vi "test.vi"() -> ()   [LabVIEW 2014]
uses:
  <vilib>/measure/maresamp.llb/Align two Waveforms (continuous).vi
  <vilib>/express/express analysis/Spectral/Block/exnSpectralBlock spectral measurements peak poly.vi
  <vilib>/express/express analysis/Spectral/Block/exnSpectralBlock spectral measurements peak DDT.vi
  <vilib>/express/express analysis/Spectral/XNode/ExpressSpectralMeasurementsBlockNode.xnode
  <vilib>/measure/NI_MAPro.lvlib
panel:
  out "Phase Difference":dbl=-4.668681158228912
  in  "Upper Cut-Off 2":dbl=12500.0 caption="Upper Cut-Off"
  in  "Upper Cut-Off":dbl=15000.0
  in  "Lower Cut-Off 2":dbl=4000.0 caption="Lower Cut-Off"
  in  "Lower Cut-Off":dbl=4000.0
  out "Demodulated R(t) Signal":dynamicdata(graph)=[{"t0"=timestamp(0 s since 1904-01-01), "dt"=2.2727272727272728e-06, "Y"=array[43991 elements], "attributes"=variant("NI_ChannelName"=variant(string "Filtered (Filtered)"), "NI_OriginalChannelName"=variant(string "Filtered"))}] caption="Filtered Signal"
  out "Demodulated I(t) Signal":dynamicdata(graph)=[{"t0"=timestamp(0 s since 1904-01-01), "dt"=2.2727272727272728e-06, "Y"=array[43991 elements], "attributes"=variant("NI_ChannelName"=variant(string "Filtered (Filtered)"), "NI_OriginalChannelName"=variant(string "Filtered"))}] caption="Filtered Signal"
  out "FFT of R(t)":dynamicdata(graph)=[{"t0"=timestamp(0 s since 1904-01-01), "dt"=10.002045873019481, "Y"=array[21996 elements], "attributes"=variant("NI_ChannelName"=variant(string "Filtered (FFT - (Peak))"), "NI_OriginalChannelName"=variant(string "Filtered"))}]
  out "FFT of I(t)":dynamicdata(graph)=[{"t0"=timestamp(0 s since 1904-01-01), "dt"=10.002045873019481, "Y"=array[21996 elements], "attributes"=variant("NI_ChannelName"=variant(string "Filtered (FFT - (Peak))"), "NI_OriginalChannelName"=variant(string "Filtered"))}]
  out "Transmitted Composit Signal":waveform(dbl)(graph)={"t0"=timestamp(3 s since 1904-01-01), "dt"=2.2727272727272728e-06, "Y"=array[44000 elements], "attributes"=variant("NI_ChannelName"=variant(string "Sine"), "NI_ExpIsRelativeTime"=variant(bool TRUE), "NI_ExpStartTimeStamp"=variant(timestamp timestamp(3501202748.2762866 s since 1904-01-01)), "NI_ExpTimeStamp"=variant(timestamp timestamp(3501202751.2762866 s since 1904-01-01)), "NI_ExpXDimension"=variant(string "t"))}
  in  "I(t) Frequency":dbl=7000.0 caption="Frequency"
  in  "I(t) Amplitude":dbl=1.0 caption="Amplitude"
  in  "R(t) Frequency":dbl=5000.0 caption="Frequency"
  in  "R(t) Amplitude":dbl=1.0 caption="Amplitude"
  out "Modulated signals":waveform(dbl)[](graph)=[{"t0"=timestamp(3 s since 1904-01-01), "dt"=2.2727272727272728e-06, "Y"=array[44000 elements], "attributes"=variant("NI_ChannelName"=variant(string "Sine"), "NI_ExpIsRelativeTime"=variant(bool TRUE), "NI_ExpStartTimeStamp"=variant(timestamp timestamp(3501202748.2762866 s since 1904-01-01)), "NI_ExpTimeStamp"=variant(timestamp timestamp(3501202751.2762866 s since 1904-01-01)), "NI_ExpXDimension"=variant(string "t"))}, {"t0"=timestamp(3 s since 1904-01-01), "dt"=2.2727272727272728e-06, "Y"=array[44000 elements], "attributes"=variant("NI_ChannelName"=variant(string "Sine"), "NI_ExpIsRelativeTime"=variant(bool TRUE), "NI_ExpStartTimeStamp"=variant(timestamp timestamp(3501202748.2762866 s since 1904-01-01)), "NI_ExpTimeStamp"=variant(timestamp timestamp(3501202751.2762866 s since 1904-01-01)), "NI_ExpXDimension"=variant(string "t"))}]
  out "Carrier":waveform(dbl)[](graph)=[{"t0"=timestamp(3 s since 1904-01-01), "dt"=2.2727272727272728e-06, "Y"=array[44000 elements], "attributes"=variant("NI_ChannelName"=variant(string "Sine"), "NI_ExpIsRelativeTime"=variant(bool TRUE), "NI_ExpStartTimeStamp"=variant(timestamp timestamp(3501202748.2762866 s since 1904-01-01)), "NI_ExpTimeStamp"=variant(timestamp timestamp(3501202751.2762866 s since 1904-01-01)), "NI_ExpXDimension"=variant(string "t"))}, {"t0"=timestamp(3 s since 1904-01-01), "dt"=2.2727272727272728e-06, "Y"=array[44000 elements]}]
  in  "Carrier Amplitude":dbl=1.0 caption="Amplitude"
  in  "Carrier Frequency":dbl=10000.0 caption="Frequency"
  in  "Carrier Amplitude 2":dbl=1.0 caption="Amplitude"
  in  "Carrier Frequency 2":dbl=10000.0 caption="Frequency"
  in  "stop 2":bool
  out "data":dynamicdata(graph)=[{"t0"=timestamp(3501202754.2033076 s since 1904-01-01), "dt"=1.1109999999999994e-05, "Y"=array[9000 elements], "attributes"=variant("NI_ChannelName"=variant(string "Voltage"), "NI_UnitDescription"=variant(string "Volts"))}] caption="Received Signal"
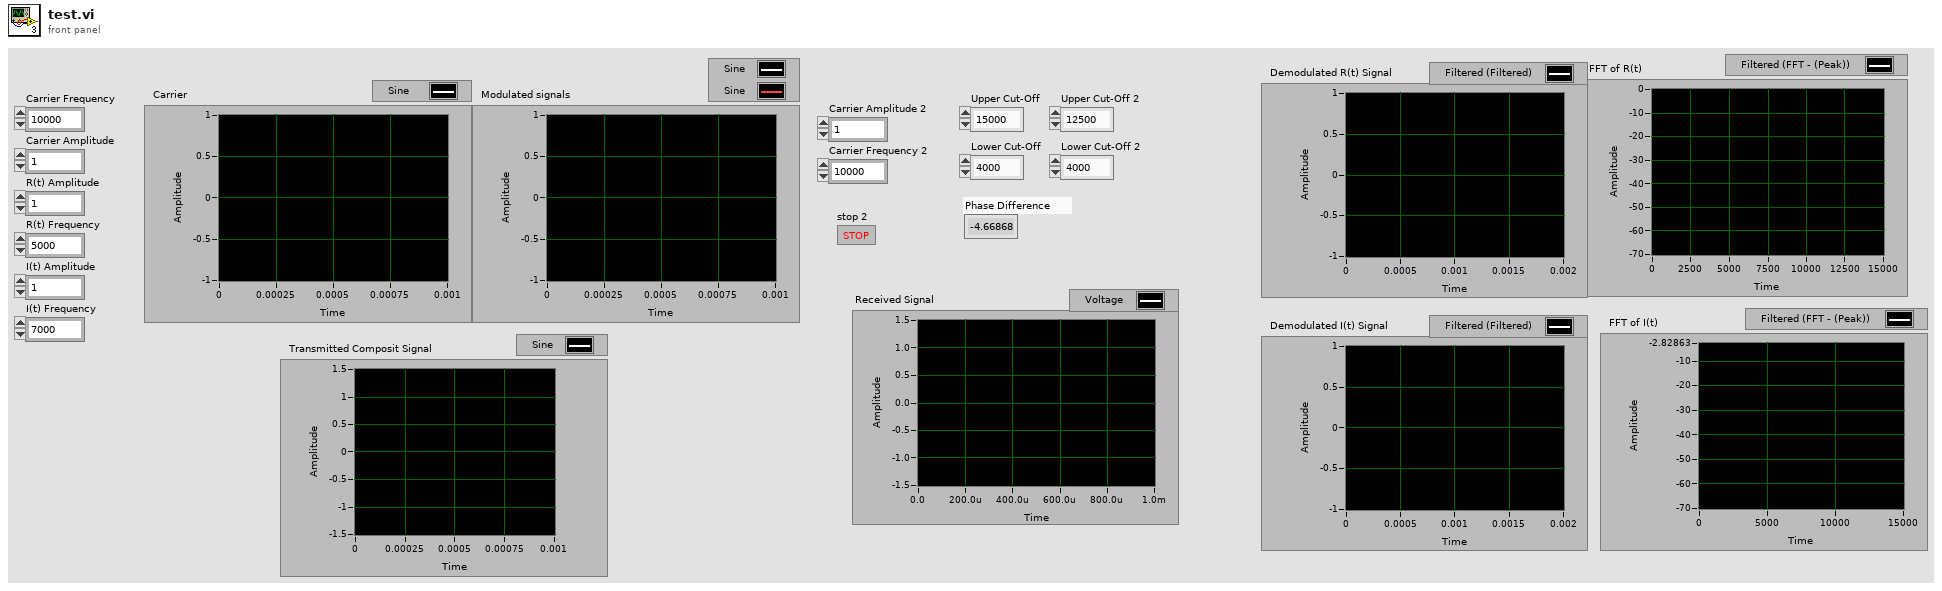
[diagram p1: front panel]
types:
  T1 = cluster{"averaging mode":u16, "weighting mode":u16, "number of averages":u32}
  T2 = cluster{"dB On (F)":bool, "unwrap phase (F)":bool, "convert to degree (F)":bool}
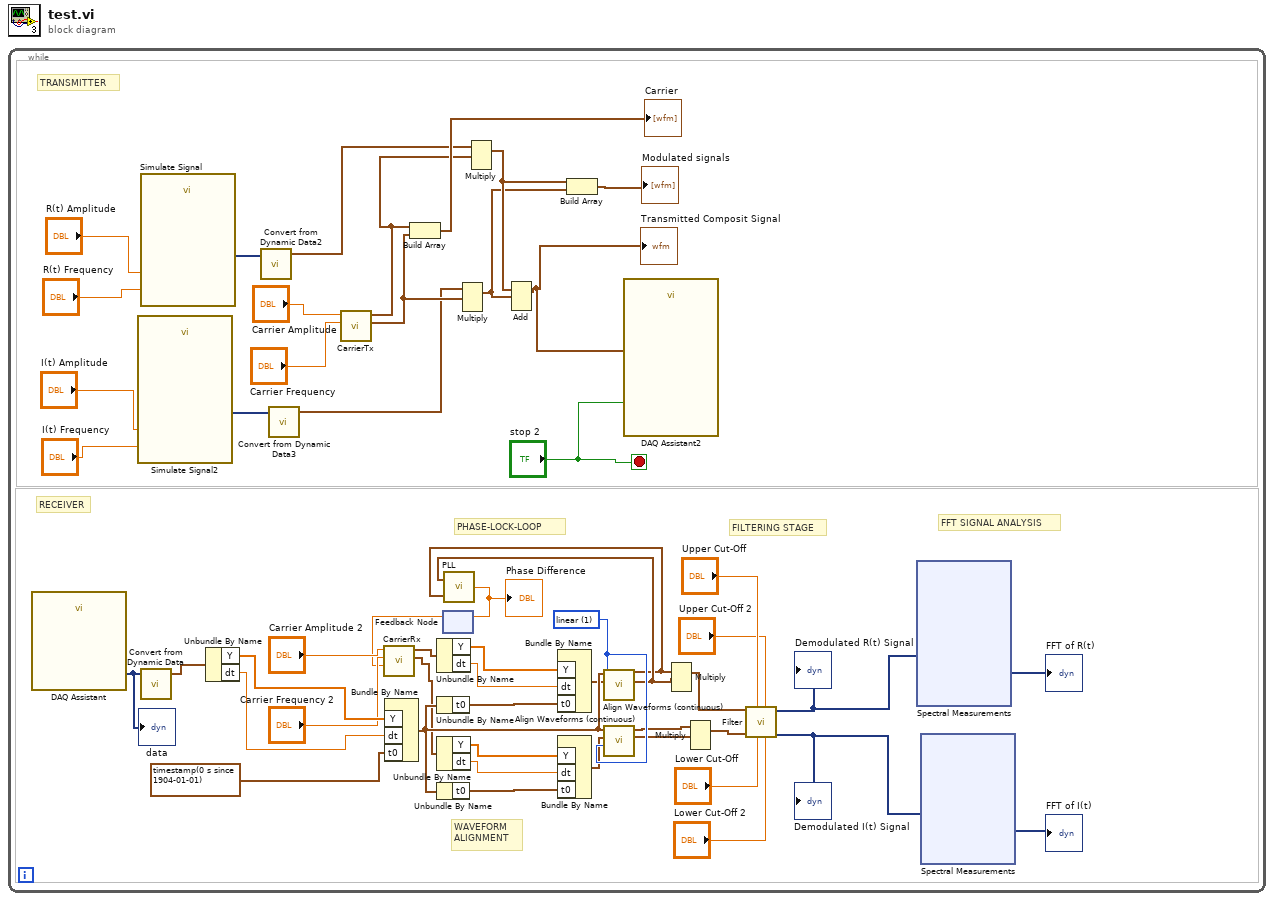
[diagram p0: block diagram]
diagram:
  n1 = while {
    stop <- "stop 2" stop-if-true
    w43 = u16 1 items=["coerce", "linear", "spline", "FIR filter"] ("interpolation mode")
    # "FFT SIGNAL ANALYSIS"
    # "FILTERING STAGE"
    # "PHASE-LOCK-LOOP"
    # "WAVEFORM\nALIGNMENT"
    # "RECEIVER"
    # "TRANSMITTER"
    n2 = call "DAQ Assistant"() -> ("data"=w53:dynamicdata)  [unwired: 17 in, 2 out]
    "data" <- w53
    n3 = call "Simulate Signal2"("Frequency"="I(t) Frequency", "Amplitude"="I(t) Amplitude") -> ("Sine"=w34:dynamicdata)  [unwired: 12 in, 1 out]
    n4 = call "Simulate Signal"("Frequency"="R(t) Frequency", "Amplitude"="R(t) Amplitude") -> ("Sine"=w39:dynamicdata)  [unwired: 12 in, 1 out]
    n5 = call "Convert from Dynamic Data"("Dynamic Data Type"=w53) -> ("Waveform"=w8:waveform(dbl))  [unwired: 3 in]
    n6 = Unbundle By Name(w8) -> ("Y"=w51:dbl[], "dt"=w50:dbl)
    n7 = call "Convert from Dynamic Data2"("Dynamic Data Type"=w39) -> ("Waveform"=w38:waveform(dbl))  [unwired: 3 in]
    n8 = call "Convert from Dynamic Data3"("Dynamic Data Type"=w34) -> ("Waveform"=w31:waveform(dbl))  [unwired: 3 in]
    n9 = call "CarrierTx.vi"("Carrier Frequency"="Carrier Frequency", "Carrier Amplitude"="Carrier Amplitude") -> ("I(t) Carrier"=w32:waveform(dbl), "R(t) Carrier"=w37:waveform(dbl))  [unwired: 8 in]
    n10 = Bundle By Name("Y"=w51, "dt"=w50, "t0"=timestamp(0 s since 1904-01-01)) -> (w44:waveform(dbl))  [unwired: 1 in]
    n11 = Build Array(w37, w32) -> (→"Carrier":waveform(dbl)[])
    n12 = Unbundle By Name(w44) -> ("t0"=w47:timestamp)
    n13 = Unbundle By Name(w44) -> ("t0"=w45:timestamp)
    n14 = feedback #1() -> (w18:dbl)  [unwired: 1 in]
    n15 = call "CarrierRx.vi"("Phase"=w18, "Carrier Frequency"="Carrier Frequency 2", "Carrier Amplitude"="Carrier Amplitude 2") -> ("I(t) Carrier"=w20:waveform(dbl), "R(t) Carrier"=w7:waveform(dbl))  [unwired: 7 in]
    n16 = Unbundle By Name(w7) -> ("Y"=w49:dbl[], "dt"=w48:dbl)
    n17 = Unbundle By Name(w20) -> ("Y"=w29:dbl[], "dt"=w46:dbl)
    n18 = Multiply(1:w32, 2:w31) -> (0:w24:waveform(dbl))  [unwired: 1 in, 1 out]
    n19 = Multiply(1:w37, 2:w38) -> (0:w25:waveform(dbl))  [unwired: 1 in, 1 out]
    n20 = Add(1:w24, 2:w25) -> (0:w26:waveform(dbl))  [unwired: 1 in, 1 out]
    "Transmitted Composit Signal" <- w26
    n21 = Bundle By Name("Y"=w49, "dt"=w48, "t0"=w47) -> (w27:waveform(dbl))  [unwired: 1 in]
    n22 = Bundle By Name("Y"=w29, "dt"=w46, "t0"=w45) -> (w28:waveform(dbl))  [unwired: 1 in]
    n23 = Build Array(w25, w24) -> (→"Modulated signals":waveform(dbl)[])
    n24 = call-poly <vilib>:"Align Waveforms (continuous).vi"("interpolation mode"=w43, "waveform B in"=w27, "waveform A in"=w44) -> ("waveform B out"=w6:waveform(dbl), "waveform A out"=w3:waveform(dbl))  [unwired: 6 in, 1 out]
    n25 = call "PLL.vi"("Local Oscillator"=w3, "Input Waveform"=w6) -> ("Phase Difference"=w19:dbl)  [unwired: 1 in]
    "Phase Difference" <- w19
    n26 = feedback-in #1(w19) -> ()
    n27 = call-poly <vilib>:"Align Waveforms (continuous).vi"("interpolation mode"=w43, "waveform B in"=w28, "waveform A in"=w44) -> ("waveform B out"=w5:waveform(dbl), "waveform A out"=w4:waveform(dbl))  [unwired: 6 in, 1 out]
    n28 = call "DAQ Assistant2"("data"=w26, "stop (F)"="stop 2") -> ()  [unwired: 15 in, 3 out]
    n29 = Multiply(1:w6, 2:w3) -> (0:w2:waveform(dbl))  [unwired: 1 in, 1 out]
    n30 = Multiply(1:w5, 2:w4) -> (0:w1:waveform(dbl))  [unwired: 1 in, 1 out]
    n31 = call "Filter.vi"("Lower Cut-Off 2"="Lower Cut-Off 2", "Upper Cut-Off 2"="Upper Cut-Off 2", "Lower Cut-Off"="Lower Cut-Off", "Upper Cut-Off"="Upper Cut-Off", "Input Waveform 2"=w1, "Input Waveform"=w2) -> ("Filtered Signal 2"=w15:dynamicdata, "Filtered Signal"=w16:dynamicdata)  [unwired: 4 in]
    "Demodulated I(t) Signal" <- w15
    "Demodulated R(t) Signal" <- w16
    n32 = xnode "Spectral Measurements"("Signals"=w16) -> ("FFT - (Peak)"=→"FFT of R(t)":dynamicdata)  [unwired: 1 in, 2 out]
    n33 = xnode "Spectral Measurements"("Signals"=w15) -> ("FFT - (Peak)"=→"FFT of I(t)":dynamicdata)  [unwired: 1 in, 2 out]
  }
